vi "Main.vi"() -> ()   [LabVIEW 2012]
uses:
  <vilib>/Utility/sysdir.llb/System Directory Type.ctl
panel:
  out "PSD (Todos Sensores)":cluster{dbl[], "Array out":dbl[]}[](graph)
  out "Aceleraciones":dynamicdata(graph)
  out "% de Buffer PSD":dbl
  in  "Main":T1(tab)
  out "CH2":dbl(knob) caption="A5-T7" scale=184.0..279.03 scale format="%^#_6g"
  out "CH1":dbl(knob) caption="A5-T5" scale=156.0..255.2 scale format="%^#_3g"
  out "CH3":dbl(knob) caption="A5-T8" scale=197.0..302.86 scale format="%^#_6g"
  out "CH4":dbl(knob) caption="A5-T6" scale=169.0..267.12 scale format="%^#_6g"
  out "CH0":dbl(knob) caption="A5-T4" scale=140.0..231.37 scale format="%^#_6g"
  out "Modo de Frecuencia encontrado":T2
  in  "Limites":T3(array[cluster])=[{"Sensor"="A5-T2", "F Min"=6.7, "F Max"=6.8, "Divisor"=1.0}, {"Sensor"="A5-T3", "F Min"=4.622, "F Max"=4.822, "Divisor"=1.0}, {"Sensor"="A6-T1", "F Min"=8.5, "F Max"=8.7, "Divisor"=1.0}, {"Sensor"="A6-T2", "F Min"=5.6, "F Max"=5.8, "Divisor"=1.0}, {"Sensor"="A5-T1", "F Min"=6.7, "F Max"=6.8, "Divisor"=1.0}]
  out "XXX":dbl(knob)=222.14170753618546 caption="A5-T4" scale=140.0..231.37 scale format="%^#_3g"
  in  "Sensor:":string(combo)="A5-T2"
  out "PSD":cluster{dbl[], "Array out":dbl[]}[](graph)
  out "Aceleracion":dbl(graph)
  out "Señal CH4":dbl(graph)
  out "Señal CH3":dbl(graph)
  out "Señal CH2":dbl(graph)
  out "Señal CH1":dbl(graph)
  out "Señal CH0":dbl(graph)
  in  "CH 4":cluster{"Semi-arpa":i32, "Tirante":i32}={"Semi-arpa"=5, "Tirante"=6} {"Tirante" min=1 max=14 step=1; "Semi-arpa" min=1 max=8 step=1}
  in  "CH 3":cluster{"Semi-arpa":i32, "Tirante":i32}={"Semi-arpa"=5, "Tirante"=8} {"Tirante" min=1 max=14 step=1; "Semi-arpa" min=1 max=8 step=1}
  in  "CH 2":cluster{"Semi-arpa":i32, "Tirante":i32}={"Semi-arpa"=5, "Tirante"=7} {"Tirante" min=1 max=14 step=1; "Semi-arpa" min=1 max=8 step=1}
  in  "CH 1":cluster{"Semi-arpa":i32, "Tirante":i32}={"Semi-arpa"=5, "Tirante"=5} {"Tirante" min=1 max=14 step=1; "Semi-arpa" min=1 max=8 step=1}
  in  "CH 0":cluster{"Semi-arpa":i32, "Tirante":i32}={"Semi-arpa"=5, "Tirante"=4} {"Tirante" min=1 max=14 step=1; "Semi-arpa" min=1 max=8 step=1}
  in  "Guardar Datos Tensiones":bool
  in  "Tamaño del archivo en seg":i32=120
  in  "Espectros cada ??":i32=120
  in  "Guardar Espectros":bool
  out "K":dbl[](array[numeric])
  in  "Stop Button":bool
  # "t"
  # "t"
  # "t"
  # "t"
  # "t"
  # "t"
  # "t"
  # "t"
  # "t"
  # "t"
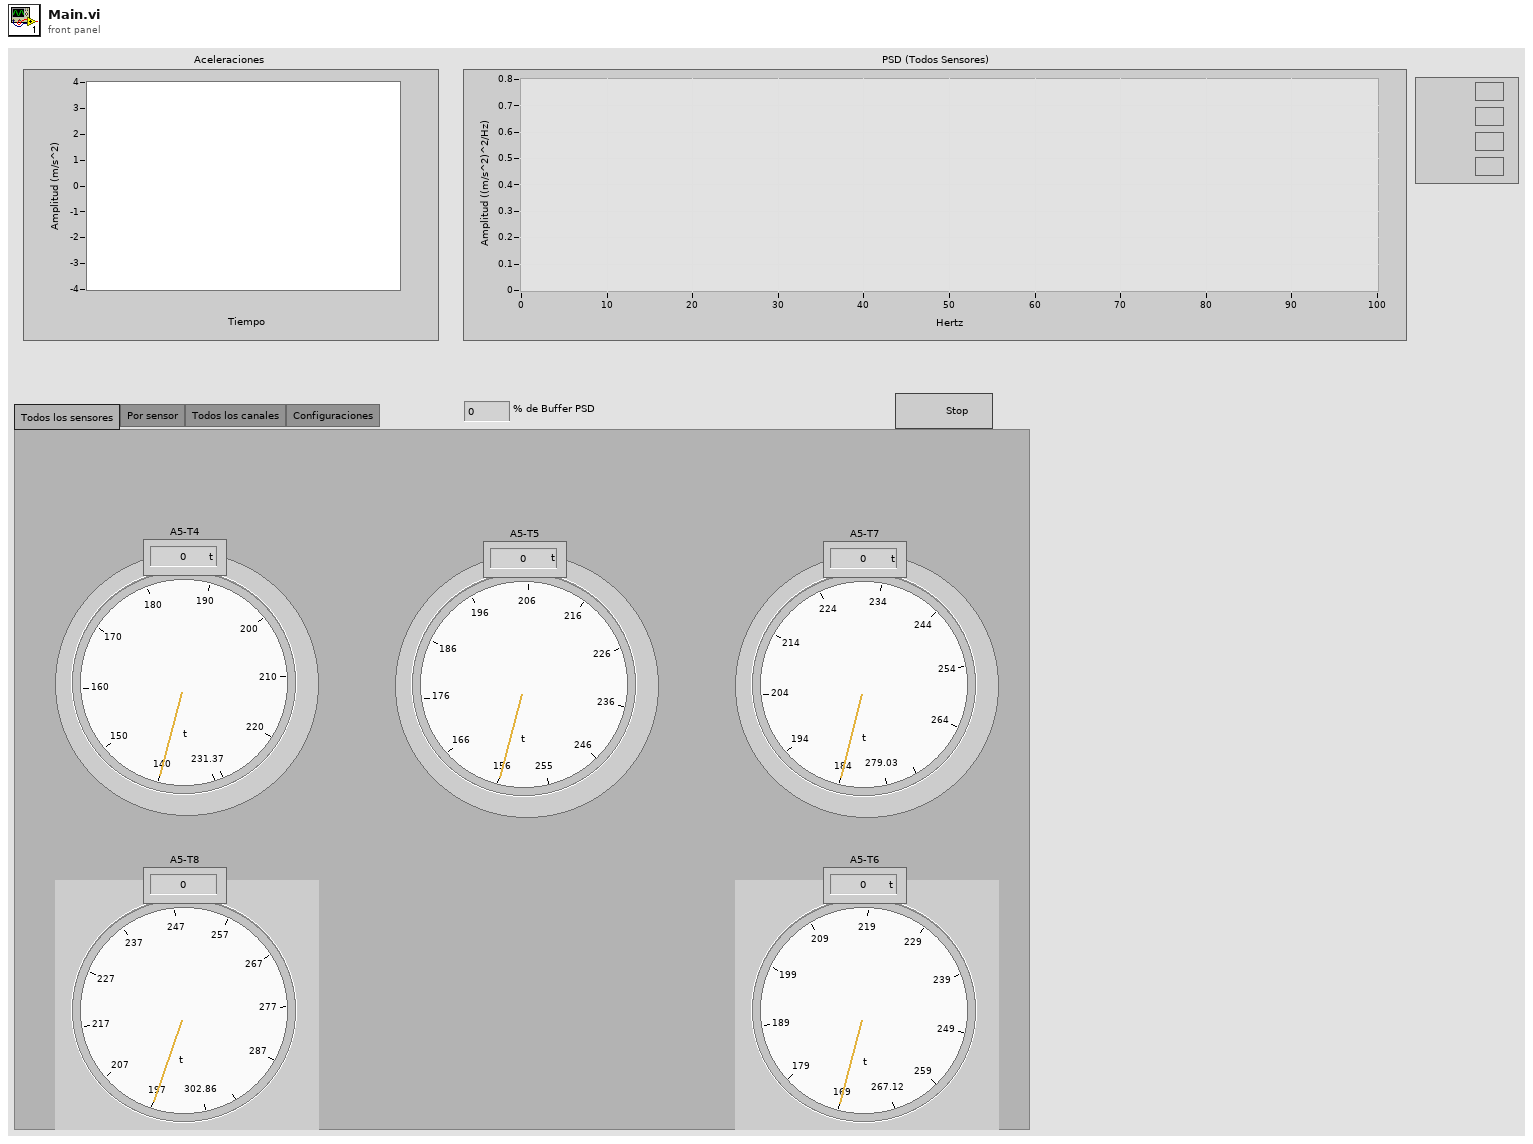
[diagram p1: front panel]
types:
  T1 = enum32{"Todos los sensores", "Por sensor", "Todos los canales", "Configuraciones"}
  T2 = cluster{"Frecuencia (Hz)  ":dbl, "Amplitud ((m/s^2)^2/Hz) ":dbl}
  T3 = cluster{"Sensor":string, "F Min":dbl, "F Max":dbl, "Divisor":dbl}[]
  T4 = cluster{string, "output cluster":cluster{"Array":cluster{"String":dbl, "Numeric Control":u32}[], "Constante K":dbl, "Frecuencia":dbl}}[]
  T5 = cluster{string, "PSD":cluster{"Frecuencia":dbl[], "Amplitud":dbl[]}, "seconds since 1Jan1904":timestamp}[]
  T6 = typedef "System Directory Type.ctl" = i32
  T7 = cluster{string, dbl, "seconds since 1Jan1904":timestamp}[]
  T8 = cluster{"Array":dbl[], "seconds since 1Jan1904":timestamp}
  T9 = cluster{"Sensor":string, dbl, "seconds since 1Jan1904":timestamp}
  T10 = cluster{"Sensor":string, "PSD":cluster{"Frecuencia":dbl[], "Amplitud":dbl[]}, "seconds since 1Jan1904":timestamp}
  T11 = cluster{"Sensor":string, "F Min":dbl, "F Max":dbl, "Divisor":dbl}
  T12 = typedef "LVCursorListTypeDef.ctl" = cluster{"Name":string, "Color":u32, "Style":u8, "Point Style":u8, "Name Visible":bool, "Allow Drag":bool, "Cursor Mode":u32, "Plot":i32, "Index":i32, "Position":cluster{"X":dbl, "Y":dbl}, "X Scale":u32, "Y Scale":u32, "Watch Plots":i32[], "Watch All Plots":bool, "Plot Area":i32, "Label Offset":cluster{"X":dbl, "Y":dbl}}[]
  T13 = cluster{"Name":string, "Color":u32, "Style":u8, "Point Style":u8, "Name Visible":bool, "Allow Drag":bool, "Cursor Mode":u32, "Plot":i32, "Index":i32, "Position":cluster{"X":dbl, "Y":dbl}, "X Scale":u32, "Y Scale":u32, "Watch Plots":i32[], "Watch All Plots":bool, "Plot Area":i32, "Label Offset":cluster{"X":dbl, "Y":dbl}}
  T14 = cluster{"Array":cluster{"String":dbl, "Numeric Control":u32}[], "Constante K":dbl, "Frecuencia":dbl}
  T15 = cluster{string, "output cluster":cluster{"Array":cluster{"String":dbl, "Numeric Control":u32}[], "Constante K":dbl, "Frecuencia":dbl}}
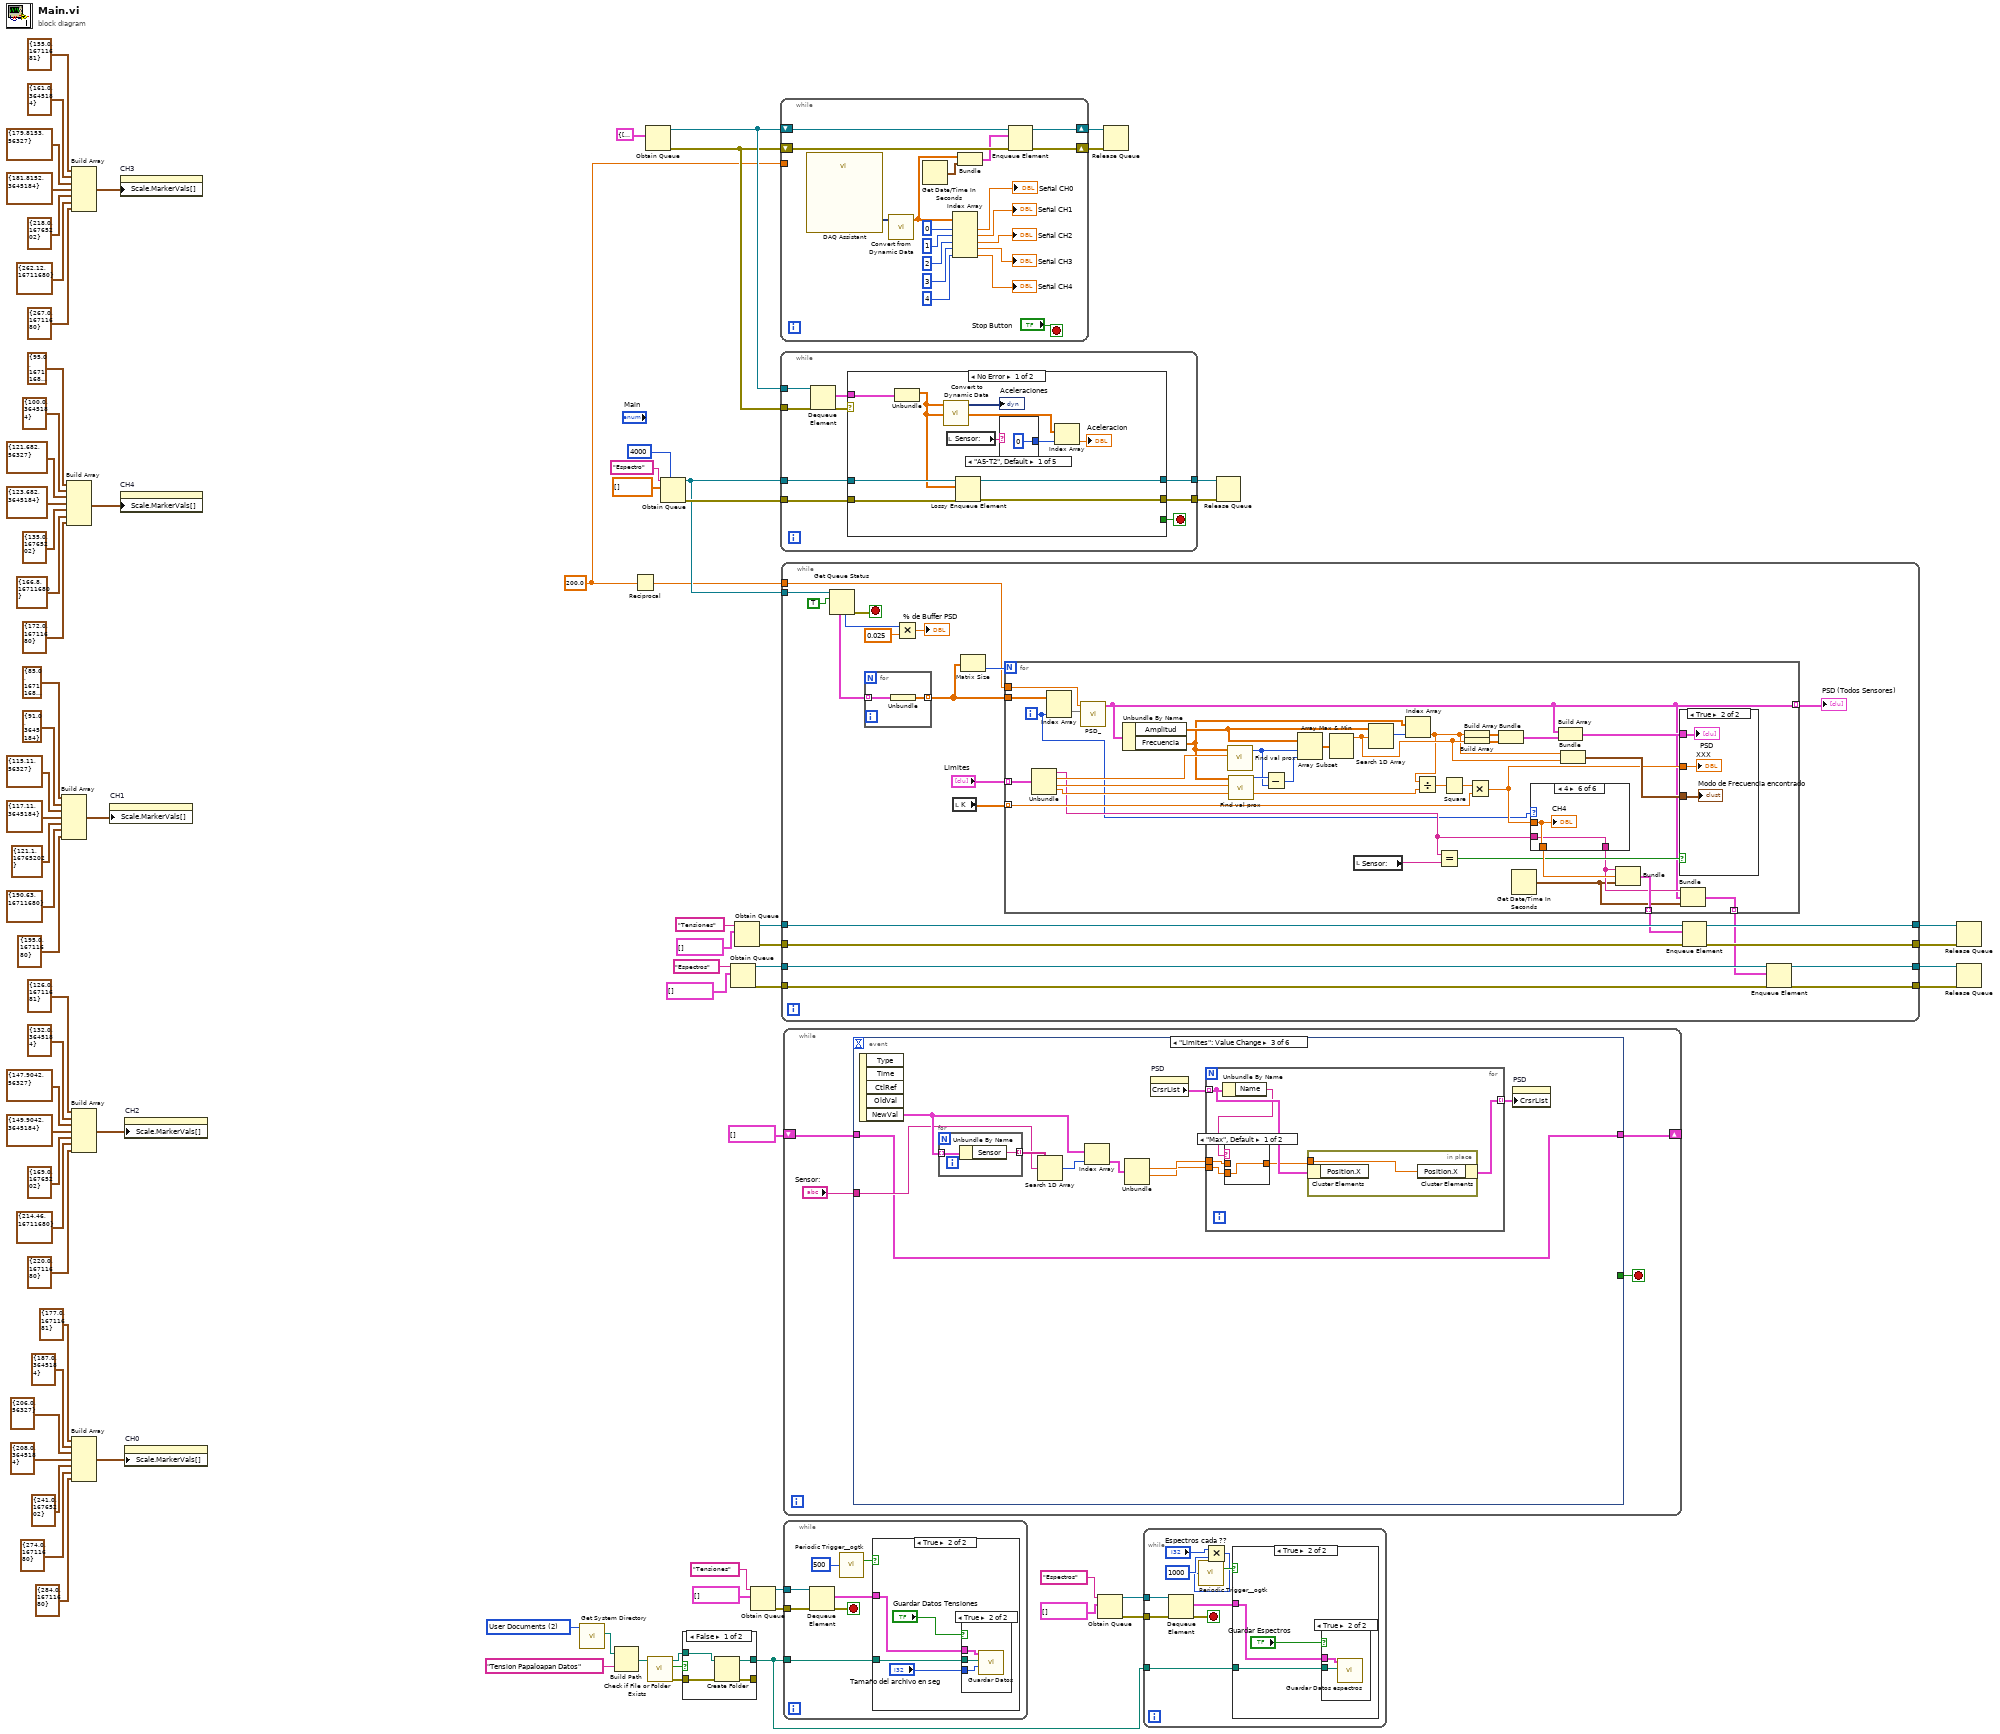
[diagram p0: block diagram]
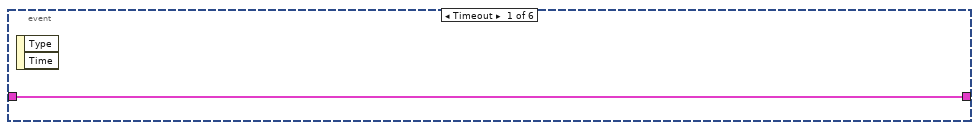
[diagram p7: hidden frame]
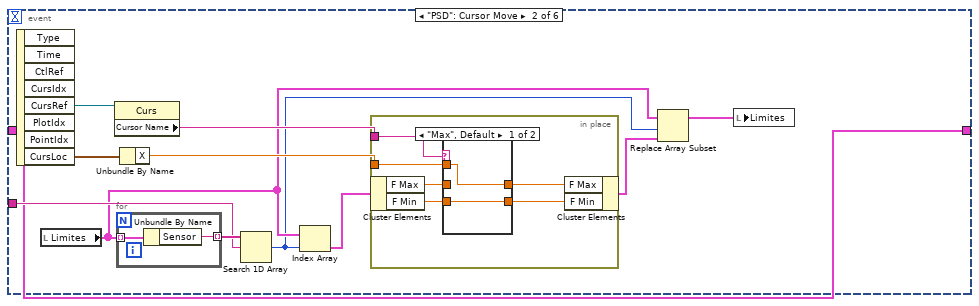
[diagram p8: hidden frame]
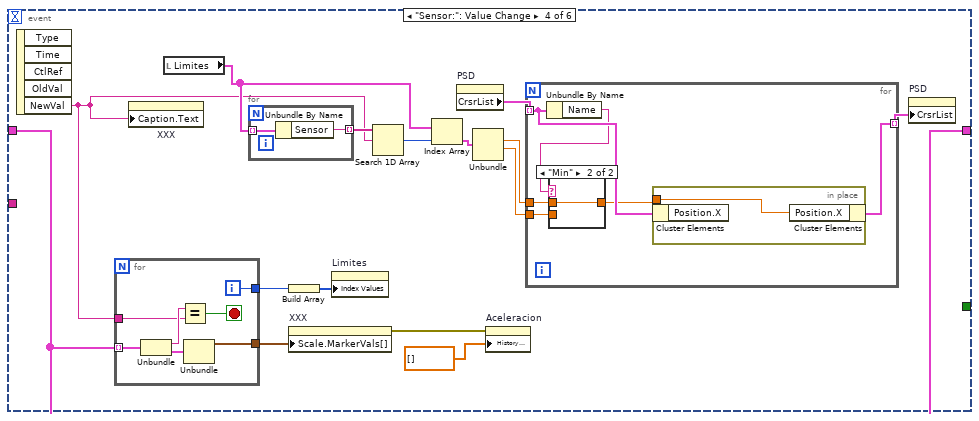
[diagram p11: hidden frame]
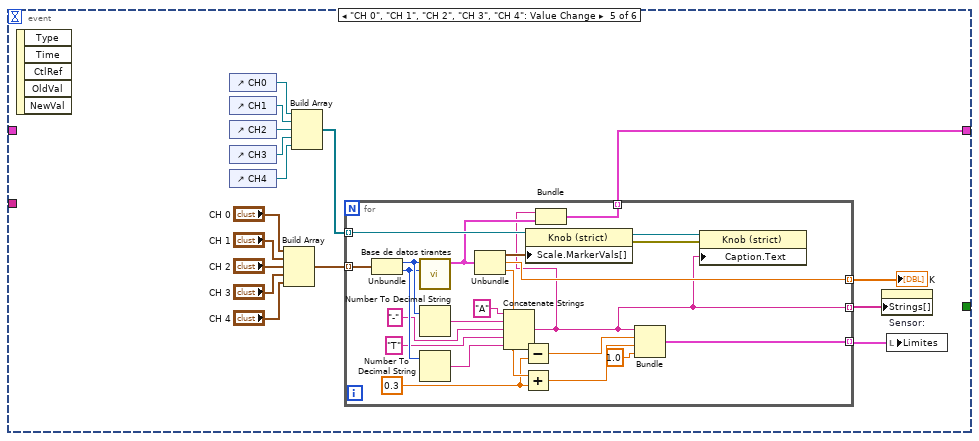
[diagram p13: hidden frame]
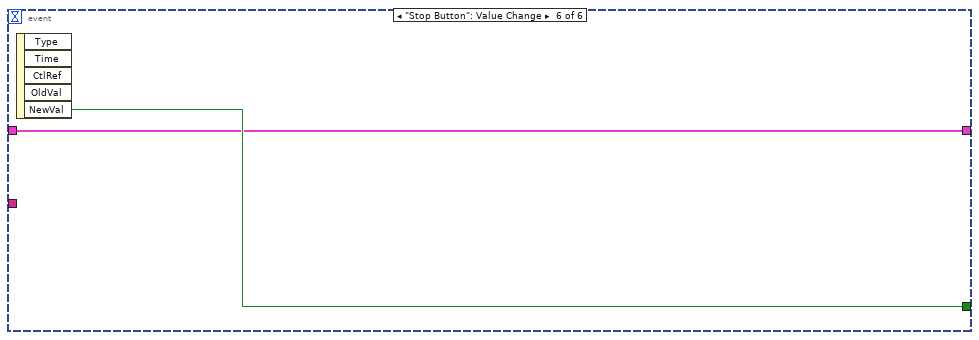
[diagram p14: hidden frame]
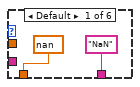
[diagram p16: hidden frame]
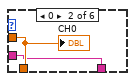
[diagram p17: hidden frame]
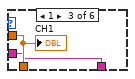
[diagram p18: hidden frame]
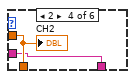
[diagram p19: hidden frame]
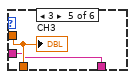
[diagram p20: hidden frame]
diagram:
  w28 = T6 2 items=["User Home"=0, "User Desktop"=1, "User Documents"=2, "User Application Data"=3, "User Preferences"=4, "User Temporary"=5, "Public Documents"=6, "Public Application Data"=7, "Public Preferences"=8, "Public Cache"=13, "System Core Libraries"=9, "System Installed Libraries"=10, "Application Files"=11, "Boot Volume Root"=12] ("system directory type")
  w70 = 200.0
  n1 = Build Array(cluster{dbl, u32} {85.0, 16711681}, cluster{dbl, u32} {91.0, 3645184}, cluster{dbl, u32} {115.11, 56327}, cluster{dbl, u32} {117.11, 3645184}, cluster{dbl, u32} {121.1, 16765202}, cluster{dbl, u32} {190.63, 16711680}, cluster{dbl, u32} {195.0, 16711680}) -> (w39:cluster{dbl, u32}[])
  n2 = Build Array(cluster{dbl, u32} {95.0, 16711681}, cluster{dbl, u32} {100.0, 3645184}, cluster{dbl, u32} {121.682, 56327}, cluster{dbl, u32} {123.682, 3645184}, cluster{dbl, u32} {135.0, 16765202}, cluster{dbl, u32} {166.8, 16711680}, cluster{dbl, u32} {172.0, 16711680}) -> (w40:cluster{dbl, u32}[])
  n3 = Build Array(cluster{dbl, u32} {155.0, 16711681}, cluster{dbl, u32} {161.0, 3645184}, cluster{dbl, u32} {179.8153, 56327}, cluster{dbl, u32} {181.8152, 3645184}, cluster{dbl, u32} {218.0, 16765202}, cluster{dbl, u32} {262.12, 16711680}, cluster{dbl, u32} {267.0, 16711680}) -> (w41:cluster{dbl, u32}[])
  n4 = Build Array(cluster{dbl, u32} {126.0, 16711681}, cluster{dbl, u32} {132.0, 3645184}, cluster{dbl, u32} {147.9042, 56327}, cluster{dbl, u32} {149.9042, 3645184}, cluster{dbl, u32} {169.0, 16765202}, cluster{dbl, u32} {214.46, 16711680}, cluster{dbl, u32} {220.0, 16711680}) -> (w38:cluster{dbl, u32}[])
  n5 = Build Array(cluster{dbl, u32} {177.0, 16711681}, cluster{dbl, u32} {187.0, 3645184}, cluster{dbl, u32} {206.0, 56327}, cluster{dbl, u32} {208.0, 3645184}, cluster{dbl, u32} {241.0, 16765202}, cluster{dbl, u32} {274.0, 16711680}, cluster{dbl, u32} {284.0, 16711680}) -> (w21:cluster{dbl, u32}[])
  n6 = property on="CH1" class="Knob (strict)"("Scale.MarkerVals[]"=w39) -> ()  [unwired: 2 in, 2 out]
  n7 = property on="CH3" class="Knob (strict)"("Scale.MarkerVals[]"=w41) -> ()  [unwired: 2 in, 2 out]
  n8 = property on="CH4" class="Knob (strict)"("Scale.MarkerVals[]"=w40) -> ()  [unwired: 2 in, 2 out]
  n9 = property on="CH2" class="Knob (strict)"("Scale.MarkerVals[]"=w38) -> ()  [unwired: 2 in, 2 out]
  n10 = property on="CH0" class="Knob (strict)"("Scale.MarkerVals[]"=w21) -> ()  [unwired: 2 in, 2 out]
  n11 = call <vilib>:"Get System Directory.vi"("system directory type"=w28) -> ("system directory"=w27:path)  [unwired: 10 in]
  n12 = Build Path(base path=w27, name or relative path="Tension Papaloapan Datos") -> (appended path=w25:path)
  n13 = Reciprocal(x=w70) -> (1/x=w71:dbl)
  n14 = Obtain Queue(element data type=T8 {"Array"=[], "seconds since 1Jan1904"=timestamp(0 s since 1904-01-01)} ("output cluster")) -> (queue out=w81:refnum<queue>, error out=w80:errorcluster)  [unwired: 4 in, 1 out]
  n15 = call <vilib>:"Check if File or Folder Exists.vi"("path"=w25) -> ("error out"=w22:errorcluster, "file or folder exists?"=w24:bool, "dup path"=w23:path)  [unwired: 8 in]
  n16 = Obtain Queue(max queue size (-1, unlimited)=4000, name (unnamed)="Espectro", element data type=dbl[] [] ("Array")) -> (queue out=w75:refnum<queue>, error out=w79:errorcluster)  [unwired: 2 in, 1 out]
  n17 = case shown="False" w24 {
    tunnel: w23 -> [w87 w89]
    tunnel: w22 -> [w86 w88]
    tunnel: [w85 w89] -> w6
    tunnel: [w84 w88] -> _
    frame False {
      n18 = Create Folder(path (use dialog)=w87, error in=w86) -> (created path=w85:path, error out=w84:errorcluster)  [unwired: 1 in, 1 out]
    }
    frame True {
    }
  }
  n19 = Obtain Queue(name (unnamed)="Espectros", element data type=T5 []) -> (queue out=w13:refnum<queue>, error out=w12:errorcluster)  [unwired: 3 in, 1 out]
  n20 = Obtain Queue(name (unnamed)="Tensiones", element data type=T7 []) -> (queue out=w34:refnum<queue>, error out=w35:errorcluster)  [unwired: 3 in, 1 out]
  n21 = Obtain Queue(name (unnamed)="Tensiones", element data type=T7 []) -> (queue out=w29:refnum<queue>, error out=w2:errorcluster)  [unwired: 3 in, 1 out]
  n22 = while {
    shift-right: [w107] -> w83
    shift-left: w81 -> [w108]
    shift-right: [w106] -> w82
    shift-left: w80 -> [w105]
    tunnel: w70 -> [_]
    stop <- "Stop Button" stop-if-true
    n23 = call "DAQ Assistant"() -> ("data"=w101:dynamicdata)  [unwired: 16 in, 3 out]
    n24 = call "Convert from Dynamic Data"("Dynamic Data Type"=w101) -> ("Array"=w100:dbl[])  [unwired: 3 in]
    n25 = Get Date/Time In Seconds() -> (seconds since 1Jan1904=w103:timestamp)
    n26 = Index Array(array=w100, index #1=0 ("index"), index #2=1 ("index"), index #3=2 ("index"), index #4=3 ("index"), index #5=4 ("index")) -> (element #1=→"Señal CH0":dbl, element #2=→"Señal CH1":dbl, element #3=→"Señal CH2":dbl, element #4=→"Señal CH3":dbl, element #5=→"Señal CH4":dbl)
    n27 = Bundle("Array"=w100, "seconds since 1Jan1904"=w103) -> (w104:T8)  [unwired: 1 in]
    n28 = Enqueue Element(queue=w108, element=w104, error in (no error)=w105) -> (queue out=w107:refnum<queue>, error out=w106:errorcluster)  [unwired: 1 in, 1 out]
  }
  n29 = while {
    tunnel: w81 -> [w117]
    tunnel: w80 -> [w116]
    tunnel: w75 -> [w112]
    tunnel: w79 -> [w111]
    tunnel: [w110] -> w77
    tunnel: [w109] -> w78
    stop <- w113 stop-if-true
    n30 = Dequeue Element(queue=w117, error in (no error)=w116) -> (element=w114:T8, error out=w115:errorcluster)  [unwired: 1 in, 2 out]
    n31 = case shown="No Error" w115 {
      tunnel: w114 -> [w123 _]
      tunnel: [_ TRUE] -> w113
      tunnel: w112 -> [w127 w134]
      tunnel: w111 -> [w125 w133]
      tunnel: [w124 w134] -> w110
      tunnel: [w126 w133] -> w109
      frame No Error {
        n32 = Unbundle(w123) -> ("Array"=w119:dbl[])  [unwired: 1 out]
        n33 = call "Convert to Dynamic Data"("Array"=w119) -> ("Dynamic Data Type"=→"Aceleraciones":dynamicdata)  [unwired: 3 in]
        n34 = local read "Sensor:"() -> (w121:string)
        n35 = Lossy Enqueue Element(queue=w127, element=w119, error in (no error)=w125) -> (queue out=w124:refnum<queue>, error out=w126:errorcluster)  [unwired: 2 out]
        n36 = case shown="\"A5-T2\", Default" w121 {
          tunnel: [0 1 2 3 4] -> w120
          frame "A5-T2", Default {
          }
          frame "A5-T3" {
          }
          frame "A6-T1" {
          }
          frame "A6-T2" {
          }
          frame "A5-T1" {
          }
        }
        n37 = Index Array(array=w119, index=w120) -> (element=→"Aceleracion":dbl)
      }
      frame Error {
      }
    }
  }
  n38 = while {
    tunnel: w75 -> [w158]
    tunnel: w71 -> [w149]
    tunnel: w34 -> [w146]
    tunnel: w35 -> [w145]
    tunnel: [w143] -> w32
    tunnel: [w142] -> w33
    tunnel: w13 -> [w139]
    tunnel: w12 -> [w138]
    tunnel: [w141] -> w10
    tunnel: [w140] -> w9
    stop <- w157 stop-if-true
    n39 = Get Queue Status(queue=w158, return elements? (F)=TRUE) -> (error out=w157:errorcluster, # elements in queue=w150:i32, elements=w156:cluster{"Array":dbl[]}[])  [unwired: 1 in, 5 out]
    n40 = for {
      tunnel: w156 -> [w210] mode=indexing
      tunnel: [w209] -> w153 mode=indexing
      n41 = Unbundle(w210) -> ("Array"=w209:dbl[])
    }
    n42 = Multiply(x=w150, y=0.025) -> (x*y=→"% de Buffer PSD":dbl)
    n43 = local read "K"() -> (w136:dbl[])
    n44 = Matrix Size(0:w153) -> (2:w154:i32)  [unwired: 1 out]
    n45 = for {
      N: w154 -> [_]
      tunnel: w149 -> [w191]
      tunnel: w153 -> [w193]
      tunnel: [w161] -> w148 mode=indexing
      tunnel: "Limites" -> [w190] mode=indexing
      tunnel: w136 -> [w177] mode=indexing
      tunnel: [w167] -> w144 mode=indexing
      tunnel: [w165] -> w137 mode=indexing
      i -> [w159]
      n46 = Unbundle(w190) -> ("Sensor"=w160:string, "F Min"=w189:dbl, "F Max"=w188:dbl, "Divisor"=w170:dbl)
      n47 = Index Array(array=w193, index (col)=w159) -> (element=w192:dbl[])  [unwired: 1 in]
      n48 = call "PSD_.vi"("Datos"=w192, "Frecuencia"=w191) -> ("PSD"=w161:cluster{"Frecuencia":dbl[], "Amplitud":dbl[]})  [unwired: 9 in]
      n49 = Unbundle By Name(w161) -> ("Amplitud"=w183:dbl[], "Frecuencia"=w181:dbl[])
      n50 = call "Find val prox.vi"("X"=w189, "Array"=w181) -> ("Index"=w185:i32)  [unwired: 9 in]
      n51 = call "Find val prox.vi"("X"=w188, "Array"=w181) -> ("Index"=w187:i32)  [unwired: 9 in]
      n52 = Subtract(x=w187, y=w185) -> (x-y=w186:i32)
      n53 = Array Subset(array=w183, index=w185, length=w186) -> (w184:dbl[])
      n54 = Array Max & Min(array=w184) -> (max value=w174:dbl)  [unwired: 3 out]
      n55 = local read "Sensor:"() -> (w176:string)
      n56 = Search 1D Array(1D array=w183, element=w174) -> (index of element=w182:i32)  [unwired: 1 in]
      n57 = Index Array(array=w181, index=w182) -> (element=w171:dbl)
      n58 = Divide(x=w171, y=w170) -> (x/y=w172:dbl)
      n59 = Equal?(x=w160, y=w176) -> (x = y?=w166:bool)
      n60 = Square(x=w172) -> (x^2=w178:dbl)
      n61 = Build Array(w171) -> (w180:dbl[])
      n62 = Build Array(w174) -> (w179:dbl[])
      n63 = Multiply(x=w178, y=w177) -> (x*y=w169:dbl)
      n64 = Bundle(w180, w179) -> (w175:cluster{dbl[], dbl[]})  [unwired: 1 in]
      n65 = Get Date/Time In Seconds() -> (seconds since 1Jan1904=w163:timestamp)
      n66 = case shown="4" w159 {
        tunnel: w169 -> [_ w200 w202 w204 w206 w208]
        tunnel: ["NaN" w199 w201 w203 w205 w207] -> w164
        tunnel: [nan w200 w202 w204 w206 w208] -> w168
        tunnel: w160 -> [_ w199 w201 w203 w205 w207]
        frame Default {
        }
        frame 0 {
          "CH0" <- w200
        }
        frame 1 {
          "CH1" <- w202
        }
        frame 2 {
          "CH2" <- w204
        }
        frame 3 {
          "CH3" <- w206
        }
        frame 4 {
          "CH4" <- w208
        }
      }
      n67 = Build Array(w161, w175) -> (w162:cluster{"Frecuencia":dbl[], "Amplitud":dbl[]}[])
      n68 = Bundle("Numeric Control"=w171, w174) -> (w173:cluster{"Numeric Control":dbl, dbl})  [unwired: 1 in]
      n69 = Bundle("Sensor"=w164, w168, "seconds since 1Jan1904"=w163) -> (w167:T9)  [unwired: 1 in]
      n70 = case shown="True" w166 {
        tunnel: w162 -> [_ w196]
        tunnel: w173 -> [_ w195]
        tunnel: w169 -> [_ w194]
        frame False {
        }
        frame True {
          "XXX" <- w194
          "PSD" <- w196
          "Modo de Frecuencia encontrado" <- w195
        }
      }
      n71 = Bundle("Sensor"=w164, "PSD"=w161, "seconds since 1Jan1904"=w163) -> (w165:T10)  [unwired: 1 in]
    }
    "PSD (Todos Sensores)" <- w148
    n72 = Enqueue Element(queue=w146, element=w144, error in (no error)=w145) -> (queue out=w143:refnum<queue>, error out=w142:errorcluster)  [unwired: 1 in, 1 out]
    n73 = Enqueue Element(queue=w139, element=w137, error in (no error)=w138) -> (queue out=w141:refnum<queue>, error out=w140:errorcluster)  [unwired: 1 in, 1 out]
  }
  n74 = while {
    shift-right: [w212] -> _
    shift-left: T4 [] -> [w211]
    stop <- w214 stop-if-true
    n75 = event shown="[2] \"Limites\": Value Change" {
      selector: _ -> [_ _ _ _ _ _]
      dyn-events: _ -> [_ _ _ _ _ _]
      timeout: _ -> [_ _ _ _ _ _]
      tunnel: [_ _ _ _ _ w333] -> w214
      tunnel: "Sensor:" -> [_ w225 w246 _ _ _]
      tunnel: [w215 w216 w240 w261 w294 w332] -> w212
      tunnel: w211 -> [w215 w216 w240 w261 _ w332]
      event Timeout {
        n76 = event-data() -> ()  [unwired: 1 in, 2 out]
      }
      event "PSD": Cursor Move {
        n77 = event-data() -> ("CursRef"=w227:refnum<vi>, "CursLoc"=w224:cluster{"X":dbl, "Y":dbl})  [unwired: 1 in, 6 out]
        n78 = local read "Limites"() -> (w220:T3)
        n79 = property class="Curs"(reference=w227) -> ("Cursor Name"=w221:string)  [unwired: 1 in, 2 out]
        n80 = for {
          tunnel: w220 -> [w239] mode=indexing
          tunnel: [w238] -> w226 mode=indexing
          n81 = Unbundle By Name(w239) -> ("Sensor"=w238:string)
        }
        n82 = Unbundle By Name(w224) -> ("X"=w223:dbl)
        n83 = Search 1D Array(1D array=w226, element=w225) -> (index of element=w219:i32)  [unwired: 1 in]
        n84 = Index Array(array=w220, index=w219) -> (element=w222:T11)
        n85 = in-place {
          in-place-border: w221 -> [w233]
          in-place-border: w223 -> [w228]
          n86 = in-place-cluster #1(w222) -> ("F Max"=w231:dbl, "F Min"=w230:dbl)
          n87 = case shown="\"Max\", Default" w233 {
            tunnel: [w235 w237] -> w232
            tunnel: w231 -> [_ w237]
            tunnel: w230 -> [w234 _]
            tunnel: [w234 w236] -> w229
            tunnel: w228 -> [w235 w236]
            frame "Max", Default {
            }
            frame "Min" {
            }
          }
          n88 = in-place-cluster #1("F Max"=w232, "F Min"=w229) -> (w218:T11)
        }
        n89 = Replace Array Subset(array=w220, new element=w218, index=w219) -> (w217:T3)
        n90 = local write "Limites"(w217) -> ()
      }
      event "Limites": Value Change {
        n91 = event-data() -> ("NewVal"=w247:T3)  [unwired: 1 in, 4 out]
        n92 = for {
          tunnel: w247 -> [w260] mode=indexing
          tunnel: [w259] -> w249 mode=indexing
          n93 = Unbundle By Name(w260) -> ("Sensor"=w259:string)
        }
        n94 = Search 1D Array(1D array=w249, element=w246) -> (index of element=w248:i32)  [unwired: 1 in]
        n95 = Index Array(array=w247, index=w248) -> (element=w244:T11)
        n96 = Unbundle(w244) -> ("F Min"=w243:dbl, "F Max"=w242:dbl)  [unwired: 2 out]
        n97 = property on="PSD" class="XYGraph (strict)"() -> ("CrsrList"=w245:T12)  [unwired: 2 in, 2 out]
        n98 = for {
          tunnel: w245 -> [w255] mode=indexing
          tunnel: w243 -> [w253]
          tunnel: w242 -> [w251]
          tunnel: [w250] -> w241 mode=indexing
          n99 = Unbundle By Name(w255) -> ("Name"=w254:string)
          n100 = case shown="\"Max\", Default" w254 {
            tunnel: w253 -> [_ w257]
            tunnel: [w256 w257] -> w252
            tunnel: w251 -> [w256 _]
            frame "Max", Default {
            }
            frame "Min" {
            }
          }
          n101 = in-place {
            in-place-border: w252 -> [w258]
            n102 = in-place-cluster #2(w255) -> ()  [unwired: 1 out]
            n103 = in-place-cluster #2("Position.X"=w258) -> (w250:T13)
          }
        }
        n104 = property on="PSD" class="XYGraph (strict)"("CrsrList"=w241) -> ()  [unwired: 2 in, 2 out]
      }
      event "Sensor:": Value Change {
        n105 = event-data() -> ("NewVal"=w264:string)  [unwired: 1 in, 4 out]
        n106 = for {
          tunnel: w261 -> [w282] mode=indexing
          tunnel: w264 -> [w280]
          tunnel: [w278] -> w262
          tunnel: [w276] -> w263
          i -> [w278]
          stop <- w279 stop-if-true
          n107 = Unbundle(w282) -> (w281:string, "output cluster"=w277:T14)
          n108 = Equal?(x=w281, y=w280) -> (x = y?=w279:bool)
          n109 = Unbundle(w277) -> ("Array"=w276:cluster{"String":dbl, "Numeric Control":u32}[])  [unwired: 2 out]
        }
        n110 = property on="XXX" class="Knob (strict)"("Caption.Text"=w264) -> ()  [unwired: 2 in, 2 out]
        n111 = local read "Limites"() -> (w267:T3)
        n112 = for {
          tunnel: w267 -> [w284] mode=indexing
          tunnel: [w283] -> w272 mode=indexing
          n113 = Unbundle By Name(w284) -> ("Sensor"=w283:string)
        }
        n114 = Build Array(w262) -> (w275:i32[])
        n115 = property on="XXX" class="Knob (strict)"("Scale.MarkerVals[]"=w263) -> (error out=w266:errorcluster)  [unwired: 2 in, 1 out]
        n116 = property on="Limites" class="Arr (strict)"("Index Values"=w275) -> ()  [unwired: 2 in, 2 out]
        n117 = Search 1D Array(1D array=w272, element=w264) -> (index of element=w271:i32)  [unwired: 1 in]
        n118 = Index Array(array=w267, index=w271) -> (element=w270:T11)
        n119 = property on="PSD" class="XYGraph (strict)"() -> ("CrsrList"=w274:T12)  [unwired: 2 in, 2 out]
        n120 = Unbundle(w270) -> ("F Min"=w268:dbl, "F Max"=w269:dbl)  [unwired: 2 out]
        n121 = property on="Aceleracion" class="WFChart (strict)"(error in=w266, "History Data"=dbl[] []) -> ()  [unwired: 1 in, 2 out]
        n122 = for {
          tunnel: w274 -> [w290] mode=indexing
          tunnel: w268 -> [w288]
          tunnel: w269 -> [w286]
          tunnel: [w285] -> w273 mode=indexing
          n123 = Unbundle By Name(w290) -> ("Name"=w289:string)
          n124 = case shown="\"Min\"" w289 {
            tunnel: w288 -> [_ w292]
            tunnel: [w291 w292] -> w287
            tunnel: w286 -> [w291 _]
            frame "Max", Default {
            }
            frame "Min" {
            }
          }
          n125 = in-place {
            in-place-border: w287 -> [w293]
            n126 = in-place-cluster #3(w290) -> ()  [unwired: 1 out]
            n127 = in-place-cluster #3("Position.X"=w293) -> (w285:T13)
          }
        }
        n128 = property on="PSD" class="XYGraph (strict)"("CrsrList"=w273) -> ()  [unwired: 2 in, 2 out]
      }
      event "CH 0", "CH 1", "CH 2", "CH 3", "CH 4": Value Change {
        n129 = event-data() -> ()  [unwired: 1 in, 5 out]
        n130 = control-ref of="CH0"() -> (w303:refnum<vi>)
        n131 = control-ref of="CH1"() -> (w302:refnum<vi>)
        n132 = control-ref of="CH2"() -> (w301:refnum<vi>)
        n133 = control-ref of="CH3"() -> (w300:refnum<vi>)
        n134 = control-ref of="CH4"() -> (w299:refnum<vi>)
        n135 = Build Array("CH 0", "CH 1", "CH 2", "CH 3", "CH 4") -> (w304:cluster{"Semi-arpa":i32, "Tirante":i32}[])
        n136 = Build Array(w303, w302, w301, w300, w299) -> (w298:refnum<vi>[])
        n137 = for {
          tunnel: w304 -> [w331] mode=indexing
          tunnel: w298 -> [w329] mode=indexing
          tunnel: [w316] -> w296 mode=indexing
          tunnel: [w315] -> w297 mode=indexing
          tunnel: [w311] -> w295 mode=indexing
          tunnel: [w310] -> w294 mode=indexing
          w327 = 0.3
          n138 = Unbundle(w331) -> ("Semi-arpa"=w326:i32, "Tirante"=w325:i32)
          n139 = call "Base de datos tirantes.vi"("Tirante"=w325, "Semi-Arpa"=w326) -> ("output cluster"=w312:T14)  [unwired: 9 in]
          n140 = Number To Decimal String(number=w326) -> (decimal integer string=w323:string)  [unwired: 1 in]
          n141 = Number To Decimal String(number=w325) -> (decimal integer string=w320:string)  [unwired: 1 in]
          n142 = Unbundle(w312) -> ("Array"=w330:cluster{"String":dbl, "Numeric Control":u32}[], "Constante K"=w315:dbl, "Frecuencia"=w328:dbl)
          n143 = Concatenate Strings("A", w323, "-", "T", w320) -> (w311:string)
          n144 = Subtract(x=w328, y=w327) -> (x-y=w319:dbl)
          n145 = Add(x=w328, y=w327) -> (x+y=w318:dbl)
          n146 = property on="Property Node" class="Knob (strict)"(reference=w329, "Scale.MarkerVals[]"=w330) -> (reference out=w314:refnum<vi>, error out=w313:errorcluster)  [unwired: 1 in]
          n147 = Bundle(w311, "output cluster"=w312) -> (w310:T15)  [unwired: 1 in]
          n148 = Bundle(w311, w319, w318, 1.0) -> (w316:cluster{string, dbl, dbl, dbl})  [unwired: 1 in]
          n149 = property on="Property Node" class="Knob (strict)"(reference=w314, error in=w313, "Caption.Text"=w311) -> ()  [unwired: 2 out]
        }
        "K" <- w297
        n150 = property on="Sensor:" class="CmbBox"("Strings[]"=w295) -> ()  [unwired: 2 in, 2 out]
        n151 = local write "Limites"(w296) -> ()
      }
      event "Stop Button": Value Change {
        n152 = event-data() -> ("NewVal"=w333:bool)  [unwired: 1 in, 4 out]
      }
    }
  }
  n153 = while {
    tunnel: w29 -> [w340]
    tunnel: w6 -> [w335]
    tunnel: w2 -> [w334]
    stop <- w339 stop-if-true
    n154 = Dequeue Element(queue=w340, error in (no error)=w334) -> (element=w338:T7, error out=w339:errorcluster)  [unwired: 1 in, 2 out]
    n155 = call <userlib>:"Periodic Trigger__ogtk.vi"("time (ms)"=u32 500) -> ("Triggered"=w336:bool)  [unwired: 12 in, 2 out]
    n156 = case shown="True" w336 {
      tunnel: w338 -> [_ w342]
      tunnel: w335 -> [_ w341]
      frame False {
      }
      frame True {
        n157 = case shown="True" "Guardar Datos Tensiones" {
          tunnel: "Tamaño del archivo en seg" -> [_ w347]
          tunnel: w342 -> [_ w346]
          tunnel: w341 -> [_ w345]
          frame False {
          }
          frame True {
            n158 = call "Guardar Datos.vi"("Intervalo de archivos (seg)"=w347, "Data folder"=w345, "Data"=w346) -> ()  [unwired: 9 in]
          }
        }
      }
    }
  }
  n159 = Obtain Queue(name (unnamed)="Espectros", element data type=T5 []) -> (queue out=w7:refnum<queue>, error out=w5:errorcluster)  [unwired: 3 in, 1 out]
  n160 = Release Queue(queue=w83, error in (no error)=w82) -> ()  [unwired: 1 in, 3 out]
  n161 = while {
    tunnel: w7 -> [w356]
    tunnel: w6 -> [w352]
    tunnel: w5 -> [w351]
    stop <- w355 stop-if-true
    n162 = Dequeue Element(queue=w356, error in (no error)=w351) -> (element=w354:T5, error out=w355:errorcluster)  [unwired: 1 in, 2 out]
    n163 = Multiply(x="Espectros cada ??", y=u32 1000 ("time (ms)")) -> (x*y=w348:u32)
    n164 = call <userlib>:"Periodic Trigger__ogtk.vi"("time (ms)"=w348) -> ("Triggered"=w353:bool)  [unwired: 12 in, 2 out]
    n165 = case shown="True" w353 {
      tunnel: w354 -> [_ w358]
      tunnel: w352 -> [_ w357]
      frame False {
      }
      frame True {
        n166 = case shown="True" "Guardar Espectros" {
          tunnel: w358 -> [_ w361]
          tunnel: w357 -> [_ w360]
          frame False {
          }
          frame True {
            n167 = call "Guardar Datos espectros.vi"("Data folder"=w360, "Data Espect"=w361) -> ()  [unwired: 10 in]
          }
        }
      }
    }
  }
  n168 = Release Queue(queue=w77, error in (no error)=w78) -> ()  [unwired: 1 in, 3 out]
  n169 = Release Queue(queue=w32, error in (no error)=w33) -> ()  [unwired: 1 in, 3 out]
  n170 = Release Queue(queue=w10, error in (no error)=w9) -> ()  [unwired: 1 in, 3 out]
